vi "Export Frames.vi"(8 "error in (no error)":errorcluster, 10 "GUID":string, 11 "Section Ref in":T3 format="%.0x") -> (0 "error out":errorcluster, 1 "Frame Settings Array":T1[](array[typedef]) {"Signals"."Byte Order" items=["Little Endian", "Big Endian"]; "Signals"."Data Type" items=["Signed", "Unsigned", "IEEE Float"]}, 2 "Frame Refs":T4[](array[typedef]) {"Signal Refs" format="%.0x"}, 3 "Section Ref out":T3 format="%.0x")   [LabVIEW 2015, in "Diagnostics Addon System Explorer.lvlib"]
uses:
  System Explorer/Diagnostics Addon System Explorer.lvlib
  <vilib>/NI Veristand/Custom Device API/Custom Device Item Ref.ctl
  Frame Signal VS References.ctl
  Shared/Frame Parameters.ctl
  Shared/Signal Parameters.ctl
  Shared/FG Action.ctl
  Shared/Get Signals.vi
  Shared/Signal Parameters FG.vi
  <vilib>/NI Veristand/Custom Device API/NI VeriStand - Get Custom Device Channel Data.vi
  <vilib>/NI Veristand/Custom Device API/NI VeriStand - Get Item Description.vi
  <vilib>/NI Veristand/Custom Device API/NI VeriStand - Get Item Property.vi
  <vilib>/NI Veristand/Custom Device API/Get Item Property (String).vi
  <vilib>/NI Veristand/Custom Device API/Get Item Property (Double).vi
  <vilib>/NI Veristand/Custom Device API/Get Item Property (U32).vi
  <vilib>/NI Veristand/Custom Device API/NI VeriStand - Set Item Property.vi
  <vilib>/NI Veristand/Custom Device API/Set Item Property (String).vi
  <vilib>/NI Veristand/Custom Device API/Set Item Property (Double).vi
  <vilib>/NI Veristand/Custom Device API/Set Item Property (U32).vi
  Shared/GUID Lookup.vi
  <vilib>/NI Veristand/Custom Device API/NI VeriStand - Get Item Data.vi
  <vilib>/NI Veristand/Custom Device Tools/Custom Device Utility Library/NI VeriStand - Search for Item by GUID.vi
  <vilib>/NI Veristand/Custom Device Tools/Custom Device Utility Library/Custom Device Utility Library.lvlib
  <vilib>/NI Veristand/Custom Device API/Custom Device API.lvlib
  Shared/Diagnostics Addon Shared.lvlib
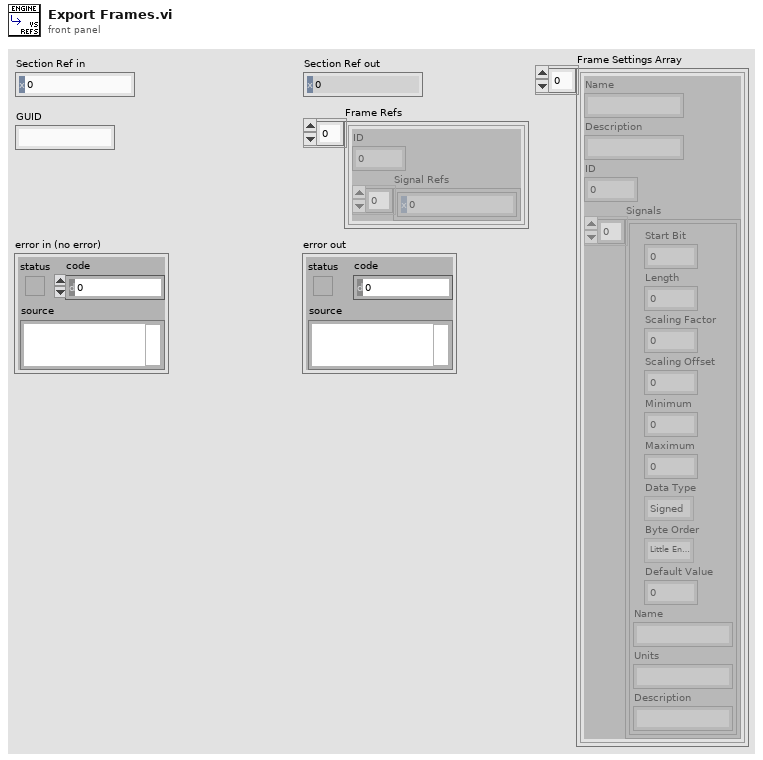
[diagram p1: front panel]
types:
  T1 = typedef "Diagnostics Addon Shared.lvlib/Frame Parameters.ctl" = cluster{"Name":string, "Description":string, "ID":u16, "Signals":T2[]}
  T2 = typedef "Diagnostics Addon Shared.lvlib/Signal Parameters.ctl" = cluster{"Start Bit":u8, "Length":u8, "Scaling Factor":dbl, "Scaling Offset":dbl, "Minimum":dbl, "Maximum":dbl, "Data Type":u32, "Byte Order":u32, "Default Value":dbl, "Name":string, "Units":string, "Description":string}
  T3 = typedef "Custom Device API.lvlib/Custom Device Item Ref.ctl" = u64
  T4 = typedef "Diagnostics Addon System Explorer.lvlib/Frame Signal VS References.ctl" = cluster{"ID":u16, "Signal Refs":T3[]}
  T5 = typedef "Diagnostics Addon System Explorer.lvlib/FG Action.ctl" = enum16{"Get", "Set"}
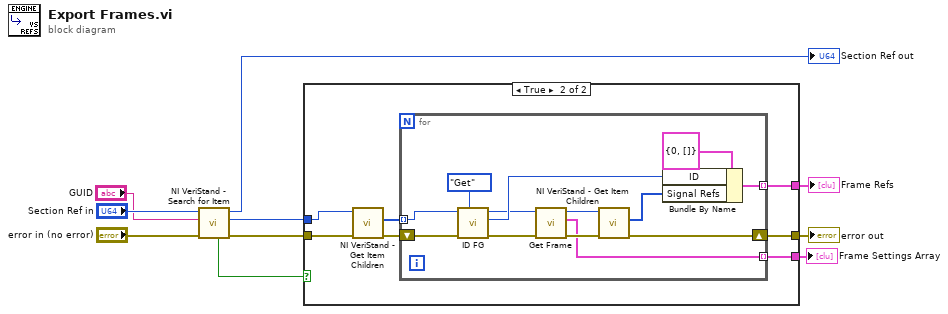
[diagram p0: block diagram]
diagram:
  n1 = call-poly <vilib>:"NI VeriStand - Search for Item.vi"("error in"="error in (no error)", "Item GUID"="GUID", "Section Ref in"="Section Ref in") -> ("error out"=w4:errorcluster, "Item Ref"=w5:T3, "Section Ref out"=→"Section Ref out":T3, "Found"=w2:bool)  [unwired: 5 in]
  n2 = case shown="True" w2 {
    tunnel: [w11 w18] -> w9
    tunnel: [_ w17] -> w8
    tunnel: w5 -> [_ w14]
    tunnel: w4 -> [w11 w13]
    tunnel: [_ w12] -> w1
    frame False {
    }
    frame True {
      n3 = call <vilib>:"NI VeriStand - Get Item Children.vi"("error in (no error)"=w13, "Item Ref in"=w14) -> ("error out"=w15:errorcluster, "Child Refs"=w16:T3[])  [unwired: 6 in, 2 out]
      n4 = for {
        shift-right: [w29] -> w18
        shift-left: w15 -> [w31]
        tunnel: w16 -> [w30] mode=indexing
        tunnel: [w25] -> w17 mode=indexing
        tunnel: [w19] -> w12 mode=indexing
        n5 = call "ID FG.vi"("Action"=FG_Action."Get", "error in (no error)"=w31, "Device Item Ref in"=w30) -> ("error out"=w23:errorcluster, "ID"=w27:u32, "Device Item Ref out"=w21:T3)  [unwired: 6 in]
        n6 = call "Get Frame.vi"("error in (no error)"=w23, "Item Ref in"=w21) -> ("error out"=w22:errorcluster, "PID In"=w19:T1, "Item Ref out"=w20:T3)  [unwired: 7 in]
        n7 = call <vilib>:"NI VeriStand - Get Item Children.vi"("error in (no error)"=w22, "Item Ref in"=w20) -> ("error out"=w29:errorcluster, "Child Refs"=w28:T3[])  [unwired: 6 in, 2 out]
        n8 = Bundle By Name(cluster=T4 {"ID"=0, "Signal Refs"=[]}, "ID"=w27, "Signal Refs"=w28) -> (w25:T4)
      }
    }
  }
  "error out" <- w9
  "Frame Refs" <- w8
  "Frame Settings Array" <- w1
